vi "SnoAutonomousMode.vi"() -> ()   [LabVIEW 2014]
uses:
  <vilib>/Rock Robotics/WPI/Solenoid/WPI_SolenoidValue.ctl
  <vilib>/Rock Robotics/WPI/RobotDrive/WPI_RobotDriveGetSetRefNum.vi
  <vilib>/Rock Robotics/Network Tables/SD Read String.vi
  <vilib>/Utility/file.llb/Read From Spreadsheet File (string).vi
  <vilib>/Rock Robotics/WPI/Solenoid/WPI_SolenoidSetEnum.vi
panel:
  out "Drive Distance (inches)":dbl
  out "Seconds for Traversal":dbl format="%0.2f"
  out "Drive Forwards 2":bool
  out "Time (sec)":dbl
  out "appended path":path
  out "File Name From DB":string
  out "Ramp Time (sec)":dbl
  out "Drive Forwards":bool
  out "Time for Distance Specified":dbl
  out "Seconds for One Meter":dbl format="%0.2f"
  out "Pot Set Point":dbl
  in  "4Bar PID gains":T1={"proportional gain (Kc)"=25.0, "integral time (Ti, min)"=0.0, "derivative time (Td, min)"=0.0}
  out "Delay Seconds":dbl
  out "Drive Speed":dbl
  out "Drive Distance Speed (0 to 0.5)":dbl
  out "Time For Drive":dbl
  out "Dleay (milliseconds)":u32
  out "Drive Distance (m)":dbl
  out "Degrees for Turn":i32
  out "Command Name":string
  out "all rows":string[][](array[string])
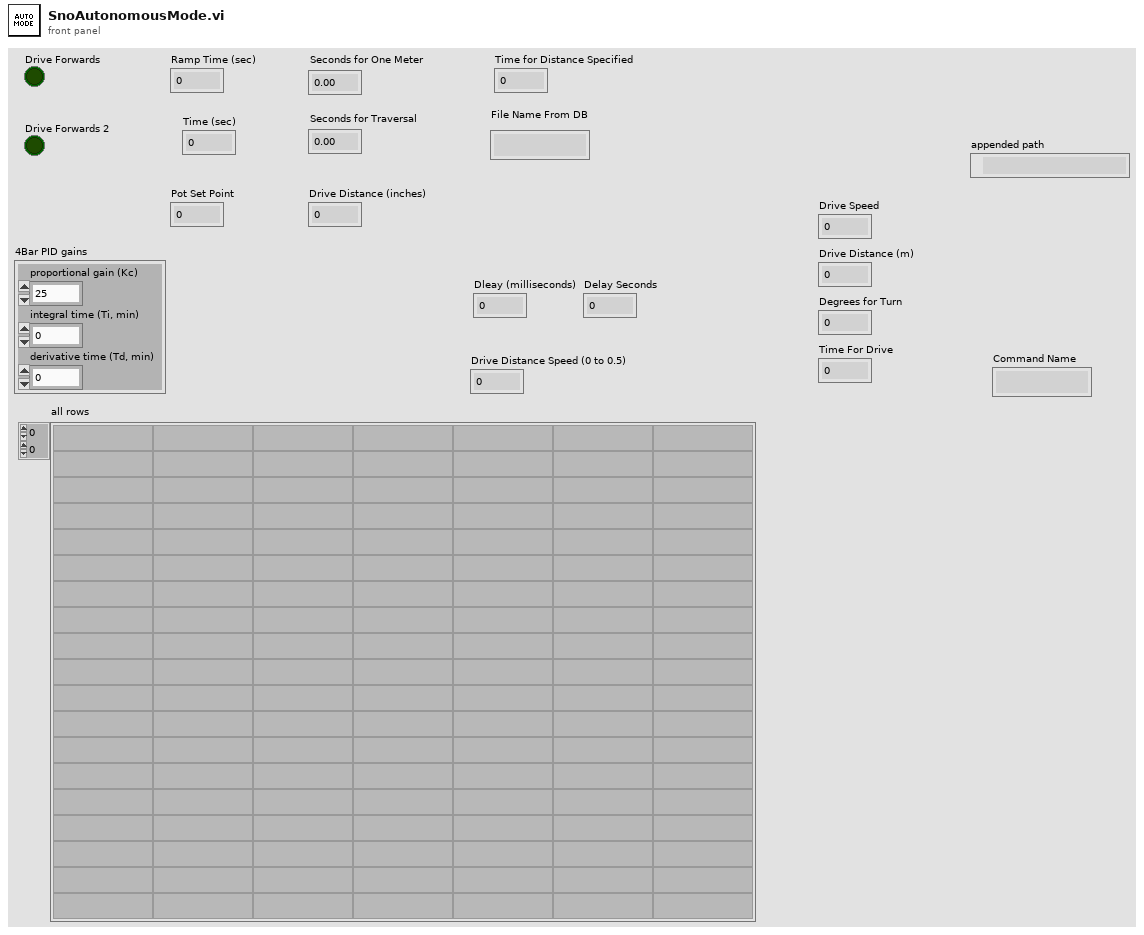
[diagram p1: front panel]
types:
  T1 = cluster{"proportional gain (Kc)":dbl, "integral time (Ti, min)":dbl, "derivative time (Td, min)":dbl}
  T2 = typedef "WPI_GyroDevRef.ctl" = cluster{"DevStatus":errorcluster, "Analog Module":T3, "Analog Channel":T4, "Offset":dbl, "Gain (VoltsPerDegree/Second)":dbl}
  T3 = typedef "FPGA_TypedefAnalogModule.ctl" = enum16{"Controller 1"}
  T4 = typedef "FPGA_AIChannel.ctl" = enum8{"AI 0", "AI 1", "AI 2", "AI 3", "AI MXP 0", "AI MXP 1", "AI MXP 2", "AI MXP 3", "Invalid"}
  T5 = typedef "WPI_PotentiometerDevRef.ctl" = cluster{"DevStatus":errorcluster, "Controller":T3, "Analog Channel":T4, "Invert Output":bool}
  T6 = typedef "WPI_MotorControlDeviceRef.ctl" = cluster{"DeviceStatus":errorcluster, "Type":T7, "PWM":cluster{"Controller":T8, "PWM Channel":T9, "DeadBand":T10}, "CAN":cluster{"Device Number":u8, "Control Mode":T11, "Semaphore":T12, "Max Vout":dbl, "TalonSRX Control Mode":T13}, "Invert":bool, "TransformRef":T14, "InvTransformRef":T14}
  T7 = typedef "WPI_MotorControlType.ctl" = enum16{"PWM", "CAN", "CANTalonSRX"}
  T8 = typedef "FPGA_TypedefDigitalModule.ctl" = enum16{"Controller 1"}
  T9 = typedef "FPGA_DIOPWMChannel.ctl" = enum8{"PWM 0", "PWM 1", "PWM 2", "PWM 3", "PWM 4", "PWM 5", "PWM 6", "PWM 7", "PWM 8", "PWM 9", "PWM MXP 0", "PWM MXP 1", "PWM MXP 2", "PWM MXP 3", "PWM MXP 4", "PWM MXP 5", "PWM MXP 6", "PWM MXP 7", "PWM MXP 8", "PWM MXP 9", "Invalid"}
  T10 = typedef "WPI_PWMDeadband.ctl" = cluster{"Name":string, "maxPositivePwm":i32, "minPositivePwm":i32, "centerPwm":i32, "maxNegativePwm":i32, "minNegativePwm":i32, "angularRange":u16}
  T11 = typedef "WPI_CANJaguar_ControlMode.ctl" = enum8{"Percent VBus", "Current", "Speed", "Position", "Voltage"}
  T12 = typedef "Semaphore RefNum" = refnum<k1>
  T13 = typedef "WPI_CANTalonSRX_APIControlMode.ctl" = enum8{"Percent VBus", "Speed", "Position", "Slave", "Unchanged / Invalid"}
  T14 = typedef "WPI_PWMTransform_ConPane.ctl" = refnum<vi>
  T15 = typedef "WPI_RobotDriveDevRef.ctl" = cluster{"DevStatus":errorcluster, "Motors[]":T6[], "Square Inputs":bool, "Max Output":dbl}
  T16 = typedef "WPI_SolenoidValue.ctl" = enum16{"Off", "On", "Forward", "Reverse"}
  T17 = typedef "WPI_SolenoidDevRef.ctl" = cluster{"DevStatus":errorcluster, "Pneumatics Control Module":u8, "Forward Solenoid Channel":T18, "Reverse Solenoid Channel":T18}
  T18 = typedef "WPI_SolenoidChannel.ctl" = enum8{"Solenoid 0", "Solenoid 1", "Solenoid 2", "Solenoid 3", "Solenoid 4", "Solenoid 5", "Solenoid 6", "Solenoid 7", "Invalid"}
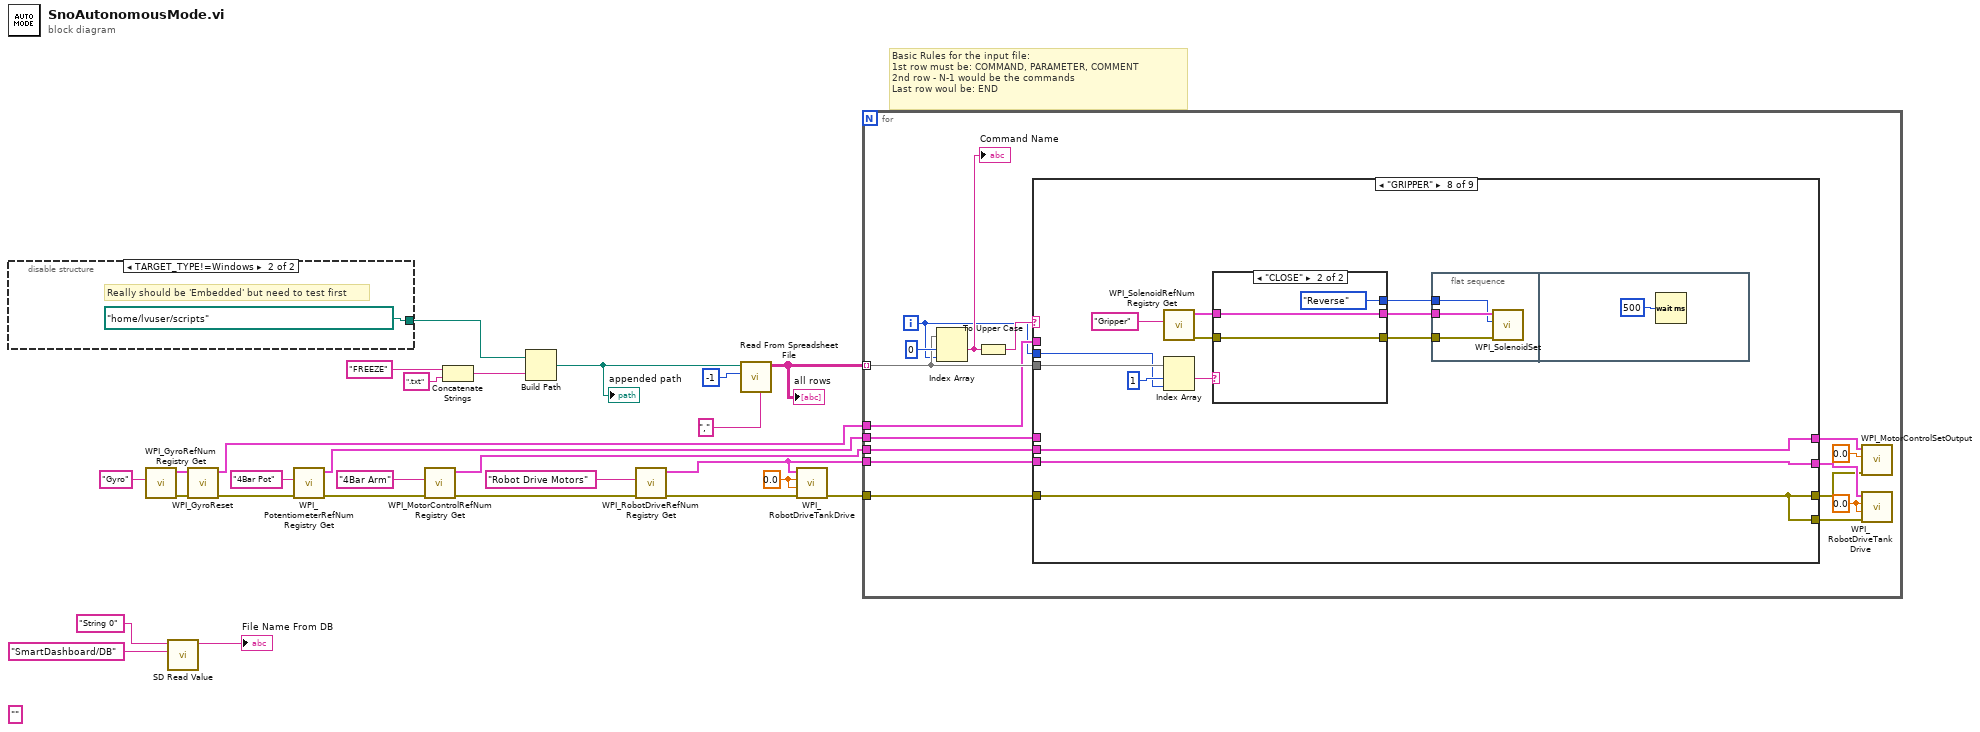
[diagram p0: block diagram]
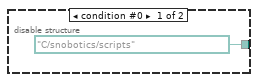
[diagram p2: hidden frame]
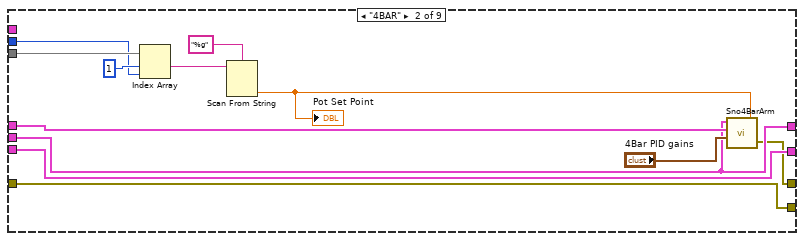
[diagram p4: hidden frame]
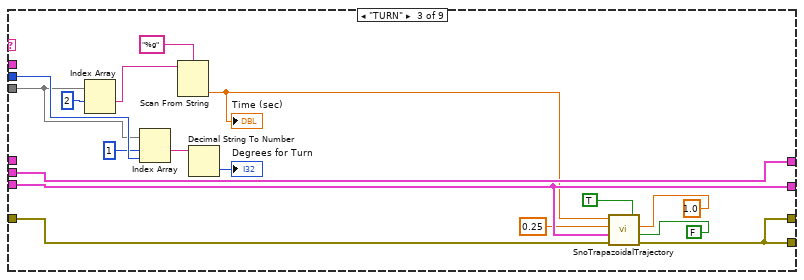
[diagram p5: hidden frame]
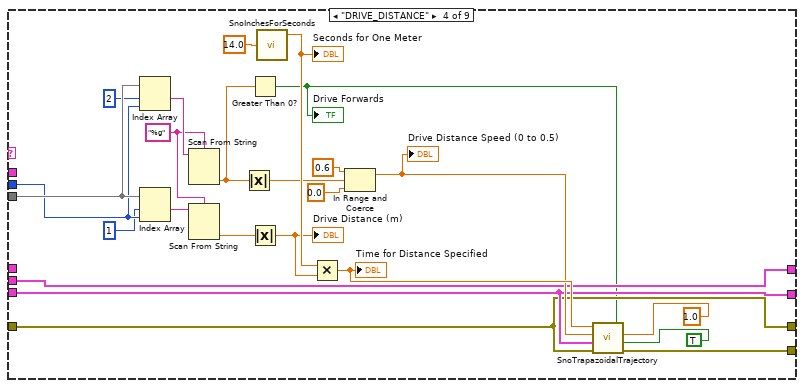
[diagram p6: hidden frame]
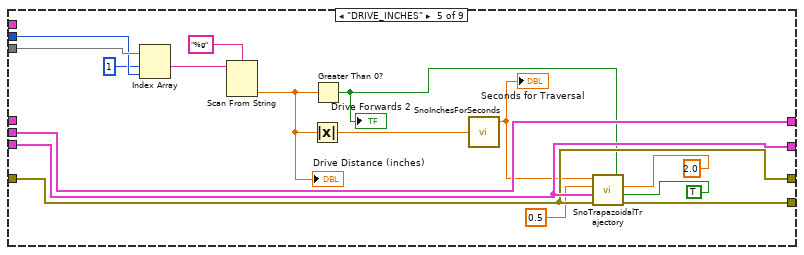
[diagram p7: hidden frame]
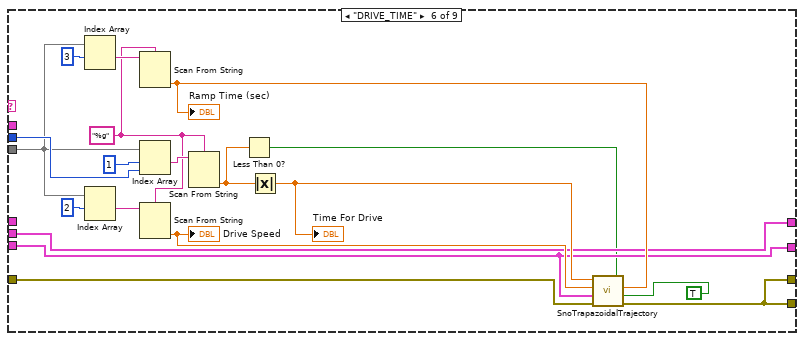
[diagram p8: hidden frame]
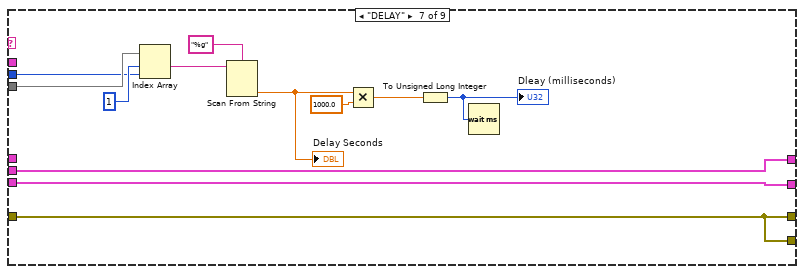
[diagram p9: hidden frame]
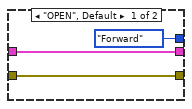
[diagram p10: hidden frame]
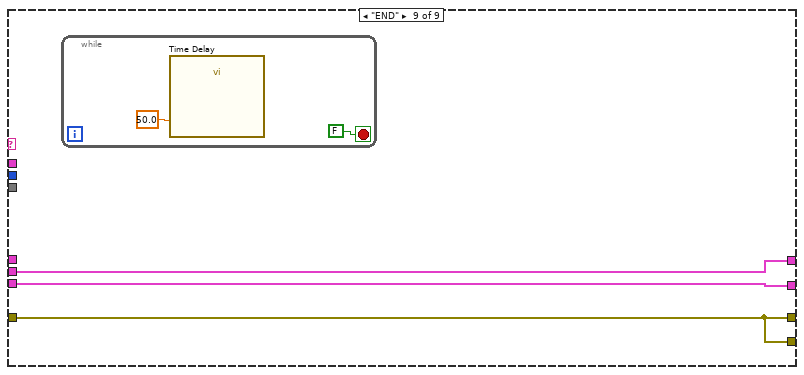
[diagram p11: hidden frame]
diagram:
  (unwired) "" ("String")
  w15 = 0.0 ("Left axis value")
  # "Basic Rules for the input file:\n1st row must be: COMMAND, PARAMETER, COMMENT\n2nd row - N-1 would be the commands\nLast row woul be: END"
  n1 = disable-structure shown="TARGET_TYPE!=Windows" {
    disable-tunnel: [path "C:/snobotics/scripts" ("path") path "/home/lvuser/scripts" ("Simulator Script Name")] -> w10
    frame condition #0 {
    }
    frame condition #1 (active) {
      # "Really should be 'Embedded' but need to test first"
    }
  }
  n2 = call <vilib>:"WPI_GyroRefNum Registry Get.vi"("refnum name"="Gyro") -> ("error out"=w26:errorcluster, "GyroDevRef"=w27:T2)  [unwired: 9 in]
  n3 = call-poly <vilib>:"SD Read Value.vi"("Table Prefix"="SmartDashboard/DB", "Name"="String 0") -> ("String"=→"File Name From DB":string)  [unwired: 7 in, 2 out]
  n4 = call <vilib>:"WPI_GyroReset.vi"("error in (no error)"=w26, "GyroDevRef"=w27) -> ("error out"=w5:errorcluster, "GyroDevRef"=w22:T2)  [unwired: 8 in]
  n5 = call <vilib>:"WPI_PotentiometerRefNum Registry Get.vi"("error in (no error)"=w5, "refnum name"="4Bar Pot") -> ("error out"=w4:errorcluster, "PotDevRef"=w18:T5)  [unwired: 8 in]
  n6 = call <vilib>:"WPI_MotorControlRefNum Registry Get.vi"("error in (no error)"=w4, "refnum name"="4Bar Arm") -> ("error out"=w3:errorcluster, "MotorControlDevRef"=w16:T6)  [unwired: 8 in]
  n7 = Concatenate Strings("FREEZE" ("string"), ".txt" ("string")) -> (w7:string)
  n8 = Build Path(base path=w10, name or relative path=w7) -> (appended path=w11:path)
  "appended path" <- w11
  n9 = call <vilib>:"WPI_RobotDriveRefNum Registry Get.vi"("error in (no error)"=w3, "refnum name"="Robot Drive Motors" ("Name")) -> ("error out"=w13:errorcluster, "RobotDriveDevRef"=w14:T15)  [unwired: 8 out]
  n10 = call-poly <vilib>:"Read From Spreadsheet File.vi"("delimiter (\\t)"="," ("delimiter (\\t)"), "number of rows (all:-1)"=-1, "file path (dialog if empty)"=w11) -> ("all rows"=w24:string[][])  [unwired: 4 in, 4 out]
  "all rows" <- w24
  n11 = call <vilib>:"WPI_RobotDriveTankDrive.vi"("error in (no error)"=w13, "Right axis value"=w15, "Left axis value"=w15, "RobotDriveDevRef"=w14) -> ("error out"=w6:errorcluster)  [unwired: 5 in, 2 out]
  n12 = for {
    tunnel: w24 -> [w44] mode=indexing
    tunnel: w22 -> [w43]
    tunnel: w14 -> [w39]
    tunnel: w18 -> [w38]
    tunnel: w16 -> [w37]
    tunnel: w6 -> [w36]
    i -> [w40]
    w33 = 0.0 ("Left axis value")
    n13 = Index Array(array=w44, index #1=0 ("index"), index #2=w40) -> (element #1=w41:string)  [unwired: 1 out]
    "Command Name" <- w41
    n14 = To Upper Case(1:w41) -> (0:w42:string)
    n15 = case shown="\"GRIPPER\"" w42 {
      tunnel: w44 -> [_ w59 w62 w101 w117 w129 w148 w161 _]
      tunnel: w40 -> [_ w58 w77 w100 w116 w136 w144 w159 _]
      tunnel: w43 -> [_ _ _ _ _ _ _ _ _]
      tunnel: w39 -> [w48 w53 w75 w83 w111 w122 w139 w158 w173]
      tunnel: w38 -> [_ w56 _ _ _ _ _ _ _]
      tunnel: w37 -> [w46 w51 w76 w80 w108 w120 w137 w156 w172]
      tunnel: w36 -> [w47 w52 w74 w81 w109 w130 w138 w157 w174]
      tunnel: [w48 w53 w75 w83 w111 w122 w139 w158 w173] -> w35
      tunnel: [w47 w52 w73 w82 w110 w121 w138 w157 w174] -> w34
      tunnel: [w46 w51 w76 w80 w108 w120 w137 w156 w172] -> w32
      tunnel: [w47 w50 w73 w81 w109 w121 w138 w157 w174] -> w30
      frame "COMMAND", Default {
      }
      frame "4BAR" {
        n16 = Index Array(array=w59, index #1=1 ("index"), index #2=w58) -> (element #1=w54:string)  [unwired: 1 out]
        n17 = Scan From String(format string="%g", input string=w54) -> (output 1=w49:dbl)  [unwired: 3 in, 3 out]
        "Pot Set Point" <- w49
        n18 = call "Sno4BarArm.vi"("Pot Set Point"=w49, "PID gains"="4Bar PID gains", "PotDevRef"=w56, "MotorControlDevRef"=w51) -> ("error out"=w50:errorcluster)  [unwired: 1 in]
      }
      frame "TURN" {
        n19 = Index Array(array=w62, index #1=2 ("index")) -> (element #1=w64:string)  [unwired: 1 in, 1 out]
        n20 = Index Array(array=w62, index #1=1 ("index"), index #2=w77) -> (element #1=w72:string)  [unwired: 1 out]
        n21 = Scan From String(format string="%g", input string=w64) -> (output 1=w61:dbl)  [unwired: 3 in, 3 out]
        "Time (sec)" <- w61
        n22 = Decimal String To Number(string=w72) -> (number=→"Degrees for Turn":i32)  [unwired: 2 in, 1 out]
        n23 = call "SnoTrapazoidalTrajectory.vi"("Straight or Turn"=FALSE, "Ramp_Up/Down_Time (sec.)"=1.0, "Drive Forward/Reverse"=TRUE, "error in"=w74, "RobotDriveDevRef"=w75, "Max Speed"=0.25, "Seconds for Traversal"=w61) -> ("error out"=w73:errorcluster)
      }
      frame "DRIVE_DISTANCE" {
        w95 = "%g" ("format string")
        n24 = Index Array(array=w101, index #1=2 ("index"), index #2=w100) -> (element #1=w97:string)  [unwired: 1 out]
        n25 = Index Array(array=w101, index #1=1 ("index"), index #2=w100) -> (element #1=w96:string)  [unwired: 1 out]
        n26 = Scan From String(format string=w95, input string=w97) -> (output 1=w86:dbl)  [unwired: 3 in, 3 out]
        n27 = Scan From String(format string=w95, input string=w96) -> (output 1=w88:dbl)  [unwired: 3 in, 3 out]
        n28 = Absolute Value(x=w86) -> (abs(x)=w87:dbl)
        n29 = Greater Than 0?(x=w86) -> (x > 0?=w79:bool)
        "Drive Forwards" <- w79
        n30 = Absolute Value(x=w88) -> (abs(x)=w89:dbl)
        "Drive Distance (m)" <- w89
        n31 = call "SnoInchesForSeconds.vi"("Inches Desired"=14.0 ("Volts Available")) -> ("Seconds for Traversal"=w92:dbl)  [unwired: 2 out]
        "Seconds for One Meter" <- w92
        n32 = Multiply(x=w92, y=w89) -> (x*y=w91:dbl)
        "Time for Distance Specified" <- w91
        n33 = In Range and Coerce(upper limit=0.6, x=w87, lower limit=0.0) -> (coerced(x)=w90:dbl)  [unwired: 1 out]
        "Drive Distance Speed (0 to 0.5)" <- w90
        n34 = call "SnoTrapazoidalTrajectory.vi"("Straight or Turn"=TRUE, "Ramp_Up/Down_Time (sec.)"=1.0, "Drive Forward/Reverse"=w79, "error in"=w81, "RobotDriveDevRef"=w83, "Max Speed"=w90, "Seconds for Traversal"=w91) -> ("error out"=w82:errorcluster)
      }
      frame "DRIVE_INCHES" {
        n35 = Index Array(array=w117, index #1=1 ("index"), index #2=w116) -> (element #1=w114:string)  [unwired: 1 out]
        n36 = Scan From String(format string="%g", input string=w114) -> (output 1=w105:dbl)  [unwired: 3 in, 3 out]
        "Drive Distance (inches)" <- w105
        n37 = Absolute Value(x=w105) -> (abs(x)=w102:dbl)
        n38 = Greater Than 0?(x=w105) -> (x > 0?=w107:bool)
        "Drive Forwards 2" <- w107
        n39 = call "SnoInchesForSeconds.vi"("Inches Desired"=w102) -> ("Seconds for Traversal"=w104:dbl)  [unwired: 2 out]
        "Seconds for Traversal" <- w104
        n40 = call "SnoTrapazoidalTrajectory.vi"("Straight or Turn"=TRUE, "Ramp_Up/Down_Time (sec.)"=2.0, "Drive Forward/Reverse"=w107, "error in"=w109, "RobotDriveDevRef"=w111, "Max Speed"=0.5, "Seconds for Traversal"=w104) -> ("error out"=w110:errorcluster)
      }
      frame "DRIVE_TIME" {
        w126 = "%g" ("format string")
        n41 = Index Array(array=w129, index #1=3 ("index")) -> (element #1=w127:string)  [unwired: 1 in, 1 out]
        n42 = Index Array(array=w129, index #1=2 ("index")) -> (element #1=w133:string)  [unwired: 1 in, 1 out]
        n43 = Scan From String(format string=w126, input string=w127) -> (output 1=w125:dbl)  [unwired: 3 in, 3 out]
        "Ramp Time (sec)" <- w125
        n44 = Index Array(array=w129, index #1=1 ("index"), index #2=w136) -> (element #1=w132:string)  [unwired: 1 out]
        n45 = Scan From String(format string=w126, input string=w133) -> (output 1=w131:dbl)  [unwired: 3 in, 3 out]
        "Drive Speed" <- w131
        n46 = Scan From String(format string=w126, input string=w132) -> (output 1=w123:dbl)  [unwired: 3 in, 3 out]
        n47 = Less Than 0?(x=w123) -> (x < 0?=w119:bool)
        n48 = Absolute Value(x=w123) -> (abs(x)=w124:dbl)
        "Time For Drive" <- w124
        n49 = call "SnoTrapazoidalTrajectory.vi"("Straight or Turn"=TRUE, "Ramp_Up/Down_Time (sec.)"=w125, "Drive Forward/Reverse"=w119, "error in"=w130, "RobotDriveDevRef"=w122, "Max Speed"=w131, "Seconds for Traversal"=w124) -> ("error out"=w121:errorcluster)
      }
      frame "DELAY" {
        n50 = Index Array(array=w148, index #1=1 ("index"), index #2=w144) -> (element #1=w143:string)  [unwired: 1 out]
        n51 = Scan From String(format string="%g", input string=w143) -> (output 1=w141:dbl)  [unwired: 3 in, 3 out]
        "Delay Seconds" <- w141
        n52 = Multiply(x=w141, y=1000.0) -> (x*y=w145:dbl)
        n53 = To Unsigned Long Integer(number=w145) -> (unsigned 32bit integer=w140:u32)
        "Dleay (milliseconds)" <- w140
        n54 = Wait (ms)(milliseconds to wait=w140) -> ()  [unwired: 1 out]
      }
      frame "GRIPPER" {
        n55 = call <vilib>:"WPI_SolenoidRefNum Registry Get.vi"("refnum name"="Gripper") -> ("error out"=w149:errorcluster, "SolenoidDevRef"=w150:T17)  [unwired: 9 in]
        n56 = Index Array(array=w161, index #1=1 ("index"), index #2=w159) -> (element #1=w155:string)  [unwired: 1 out]
        n57 = case shown="\"CLOSE\"" w155 {
          tunnel: w149 -> [w167 w169]
          tunnel: w150 -> [w168 w170]
          tunnel: [w168 w170] -> w153
          tunnel: [w167 w169] -> w152
          tunnel: [WPI_SolenoidValue."Forward" ("Value") WPI_SolenoidValue."Reverse" ("Value")] -> w151
          frame "OPEN", Default {
          }
          frame "CLOSE" {
          }
        }
        n58 = flat-sequence {
          tunnel: w153 -> [w164]
          tunnel: w152 -> [w163]
          tunnel: w151 -> [w162]
          frame #0 {
            n59 = call-poly <vilib>:"WPI_SolenoidSet.vi"("error in (no error)"=w163, "Value"=w162, "SolenoidDevRef"=w164) -> ()  [unwired: 7 in, 2 out]
          }
          frame #1 {
            n60 = Wait (ms)(milliseconds to wait=u32 500) -> ()  [unwired: 1 out]
          }
        }
      }
      frame "END" {
        n61 = while {
          stop <- FALSE stop-if-true
          n62 = call "Time Delay"("Delay Time (s)"=50.0) -> ()  [unwired: 10 in, 1 out]
        }
      }
    }
    n63 = call <vilib>:"WPI_MotorControlSetOutput.vi"("error in (no error)"=w30, "Output"=0.0, "MotorControlDevRef"=w32) -> ()  [unwired: 6 in, 3 out]
    n64 = call <vilib>:"WPI_RobotDriveTankDrive.vi"("error in (no error)"=w34, "Right axis value"=w33, "Left axis value"=w33, "RobotDriveDevRef"=w35) -> ()  [unwired: 5 in, 3 out]
  }
